vi "OME_coMD.vi"() -> ()   [LabVIEW 2012]
doc: "SciScan 1.2 160622"
uses:
  Macro Module/MacroGUI Module/Custom Controls and Typedefs/Cancel Settings.ctl
  Macro Module/MacroGUI Module/Custom Controls and Typedefs/Confirm Settings.ctl
  Custom Controls and Typedefs/Channel Parameters Cluster.ctl
  Custom Controls and Typedefs/Experiment and Experimenter.ctl
  Custom Controls and Typedefs/Objective Parameters Cluster.ctl
  Custom Controls and Typedefs/OME_MD_GUI control references.ctl
  CommonResource VIs/UI Control and Indicator properties_Commands.ctl
  SubVIs/FGV_ExclusionList_Manager_Commands.ctl
  CommonResource VIs/FormatTree&TableStyle_Commands.ctl
  GFG/GFGpathGet.vi
  <vilib>/xml/Close Reference(Node).vi
  <resource>/objmgr/DOMUserDefRef.rc
  <vilib>/xml/NI_XML.lvlib
  GFG/GFG library.lvlib
panel:
  in  "Objective Parameters":T1[](array[typedef])
  in  "Experiment Parameters":T2
  out "Parse Errors":string
  in  "Channel Parameters":T3[](array[typedef]) {"Excitation Wavelength" min=1e-07; "Emission Wavelength" min=1e-07}
  out "Selected Parameter Path":string caption="/OME/Experiment/ExperimenterRef/@ID"
  in  "Confirm":T4
  in  "Cancel":T5
  out "x-y":u32
  in  "Stop Button":bool
  in  "Refresh Button":bool
  in  "Param Value (Edit)":string caption="/OME/Experiment/ExperimenterRef/@ID"
  in  "XML 2D Array":string[][](array[string])
  in  "OME XML Parameters":string(tree)
  # "Experiment"
  # "Experimenter"
  # "Sample"
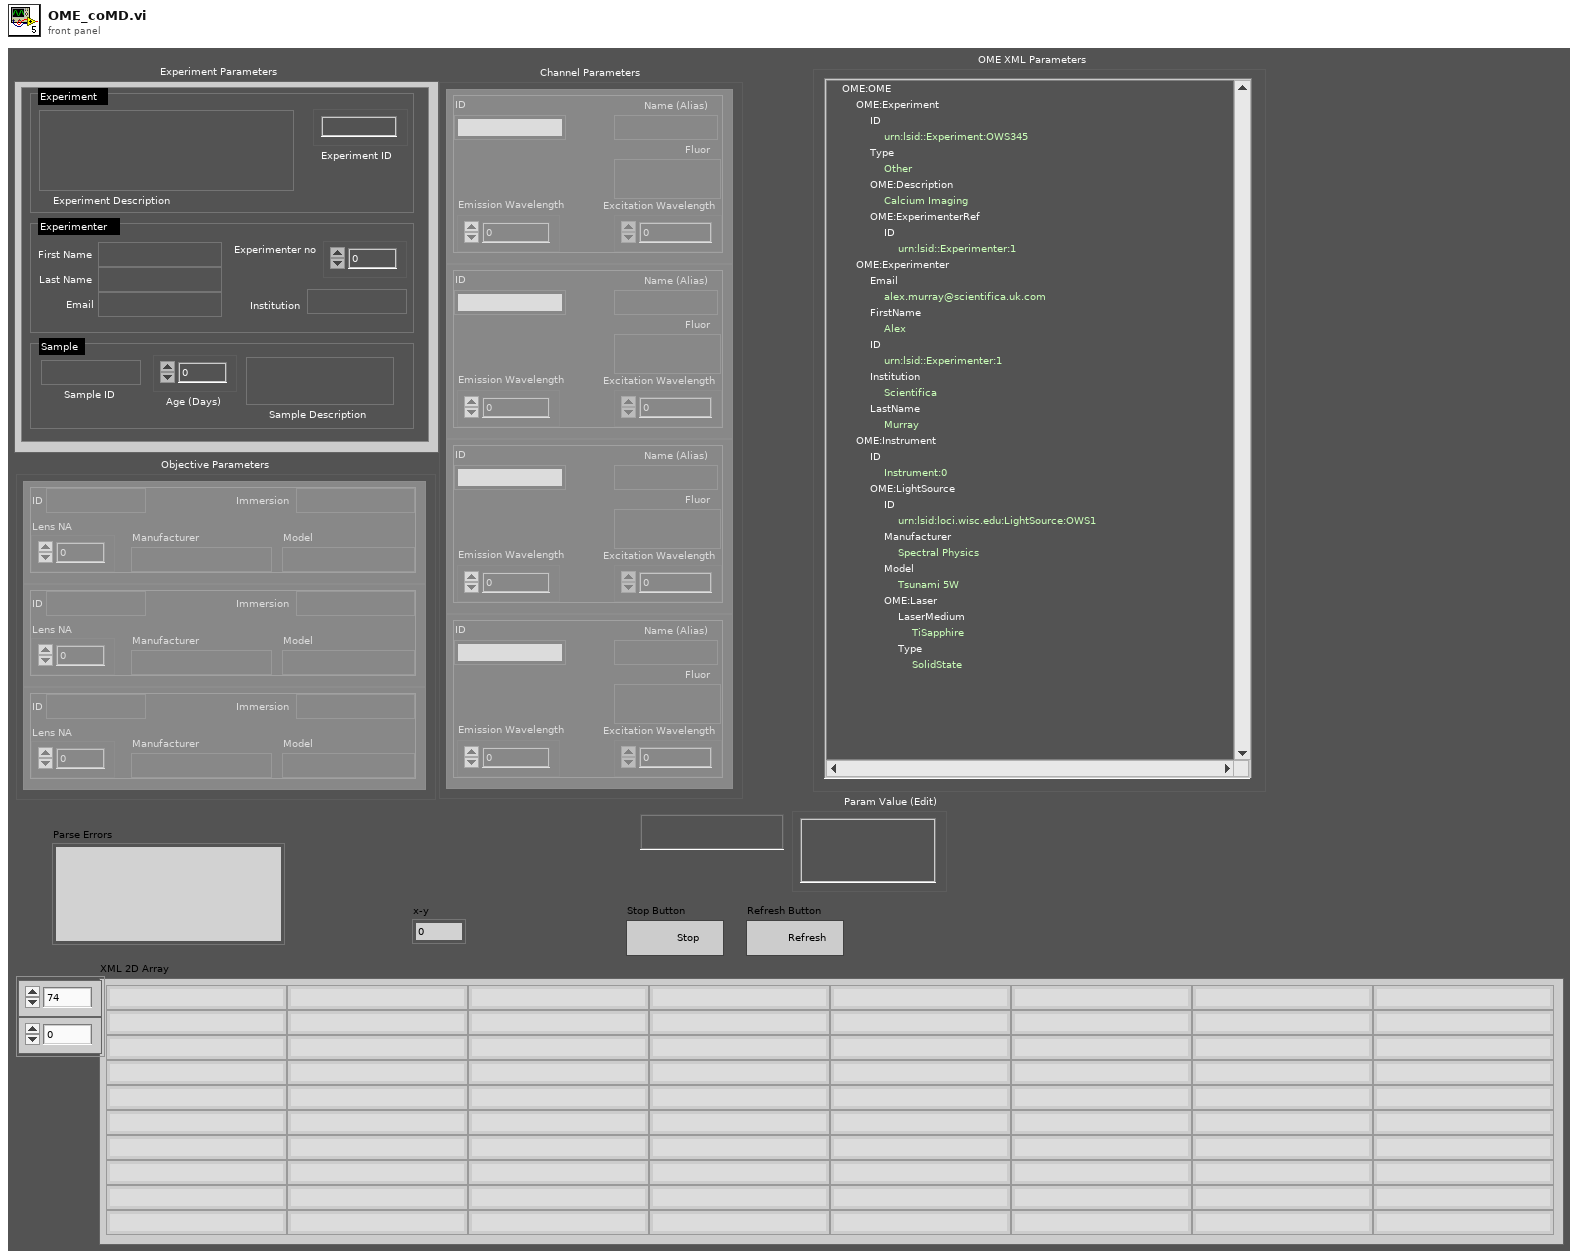
[diagram p1: front panel]
types:
  T1 = typedef "Objective Parameters Cluster.ctl" = cluster{"ID":string, "Immersion":string, "Lens NA":dbl, "Manufacturer":string, "Model":string}
  T2 = typedef "Experiment and Experimenter.ctl" = cluster{"Experimenter no":u32, "First Name":string, "Experiment ID":string, "urn:lsid: ":string, "Experiment Description":string, "Last Name":string, "Email":string, "Institution":string, "Sample ID":string, "Age (Days)":u32, "Sample Description":string}
  T3 = typedef "Channel Parameters Cluster.ctl" = cluster{"Name (Alias)":string, "ID":string, "Fluor":string, "Colour (RGBA encoded)":i32, "Emission Wavelength":dbl, "Excitation Wavelength":dbl}
  T4 = typedef "Confirm Settings.ctl" = bool
  T5 = typedef "Cancel Settings.ctl" = bool
  T6 = typedef "FGV_ExclusionList_Manager_Commands.ctl" = enum16{"Initialize(ReadCSV)", "Get", "CategorizePaths"}
  T7 = typedef "UI Control and Indicator properties_Commands.ctl" = enum16{"Enable", "Disable", "Disable and Grey", "Make Visible", "Make Invisible"}
  T8 = typedef "OME_MD_GUI control references.ctl" = cluster{"2D Array":refnum<vi>, "XML Tree":refnum<vi>, "Param Value":refnum<vi>, "Cancel":refnum<vi>, "Confirm":refnum<vi>, "Param Path":refnum<vi>, "Objective Parameters":refnum<vi>, "Experiment and Experimenter Details":refnum<vi>, "Channel Parameters":refnum<vi>}
  T9 = typedef "FormatTree&TableStyle_Commands.ctl" = enum16{"Colour Row", "Uncolour Row", "Bold Row", "Unbold Row", "Clear", "UpdateVisibleRows"}
  T10 = enum32{"Invalid", "Standard", "Closed", "Hidden", "Minimized", "Maximized"}
  T11 = typedef "eventvkey.ctl" = enum16{"ASCII", "Enter", "Return", "Shift", "Ctrl", "Alt", "Cmd", "Opt", "Caps", "NumLock", "Clear", "Break", "Up", "Down", "Left", "Right", "Insert", "Delete", "Home", "End", "PageUp", "PageDown", "Escape", "Help", "Pause", "ScrollLock", "F1", "F2", "F3", "F4", "F5", "F6", "F7", "F8", "F9", "F10", "F11", "F12", "F13", "F14", "F15", "F16", "F17", "F18", "F19", "F20", "F21", "F22", "F23", "F24", "Play", "VolumeUp", "VolumeDown", "Mute", "Two Byte Char"}
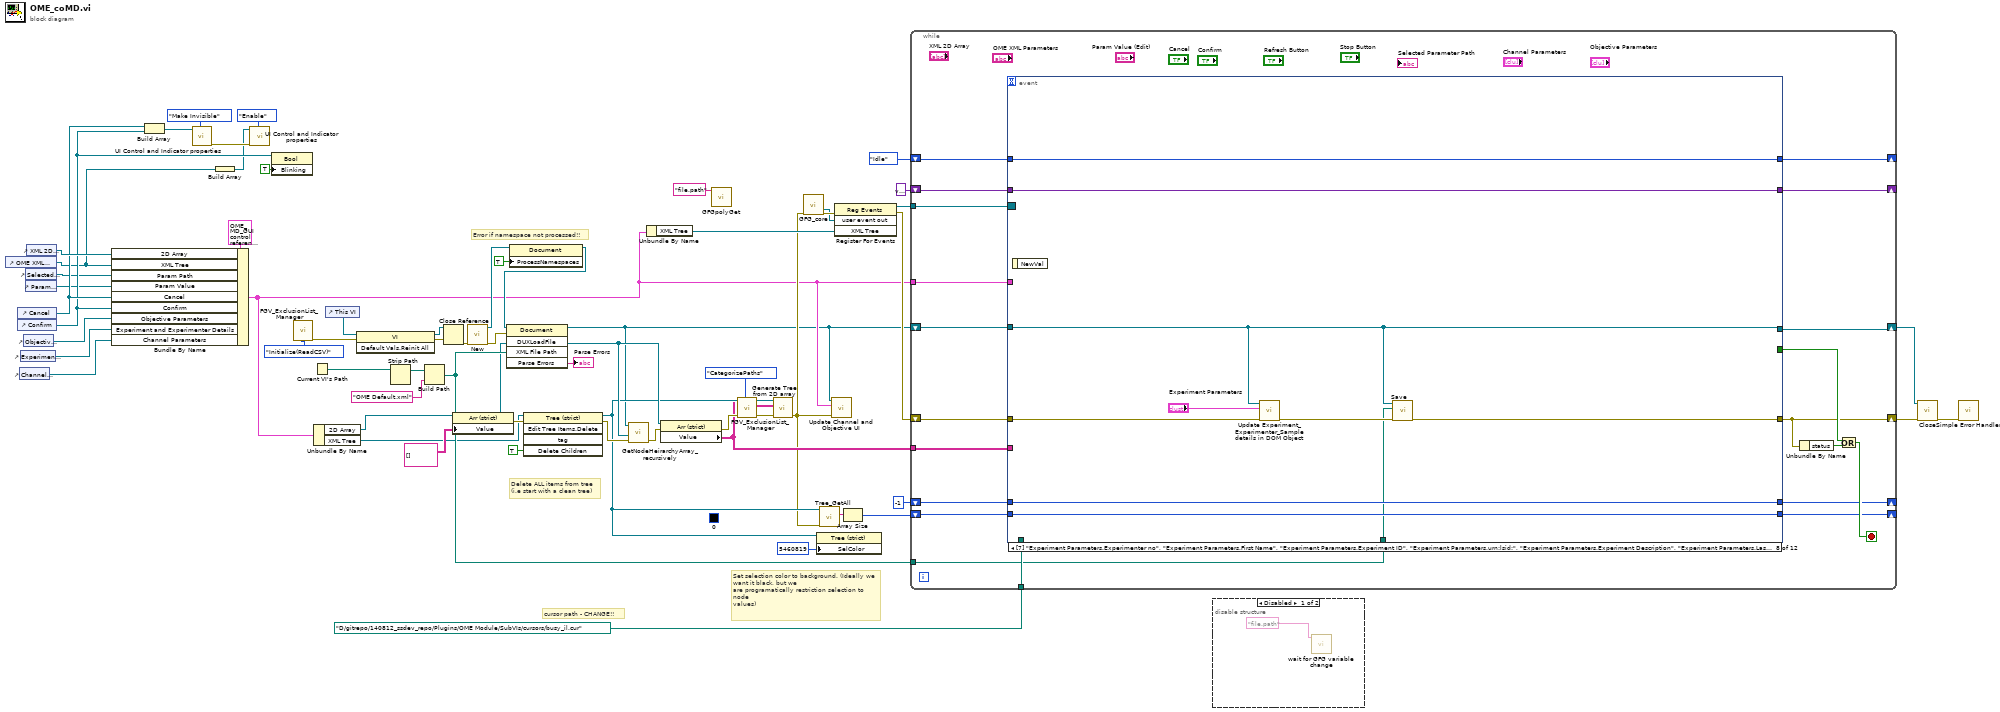
[diagram p0: block diagram]
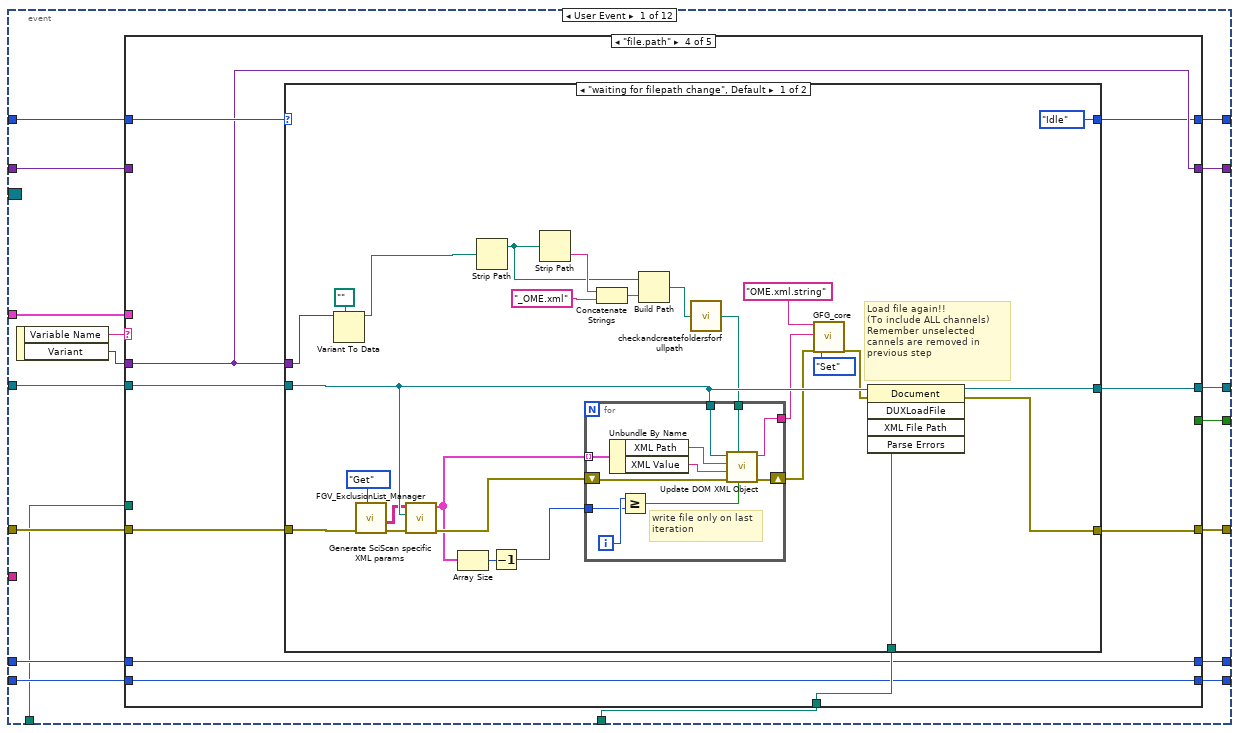
[diagram p3: hidden frame]
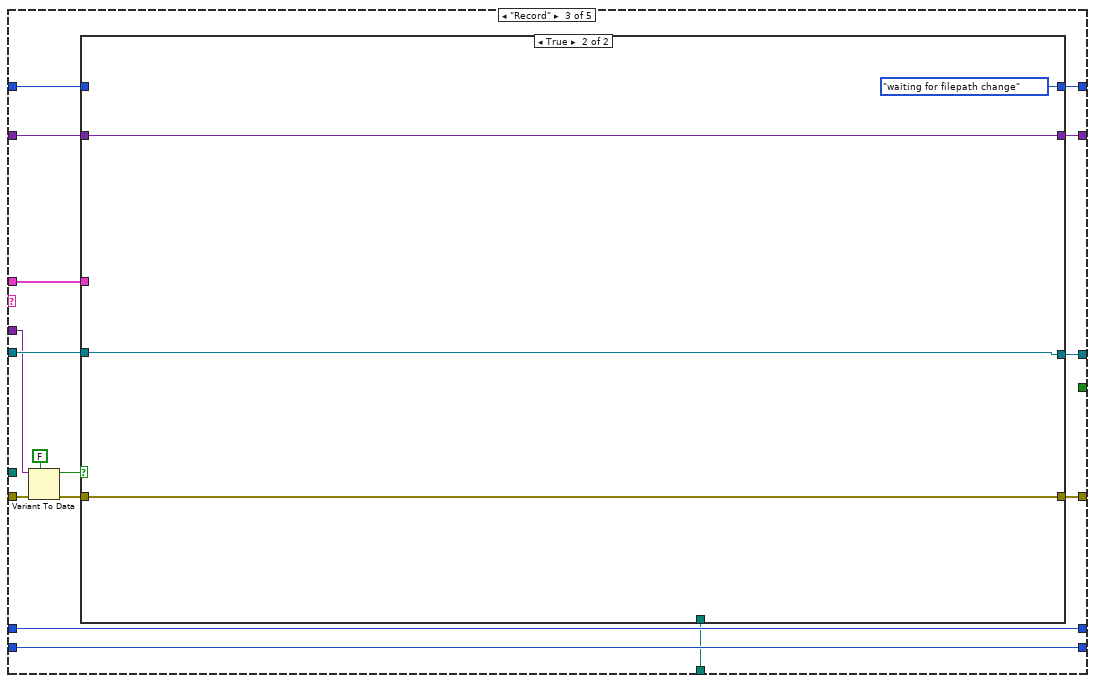
[diagram p6: hidden frame]
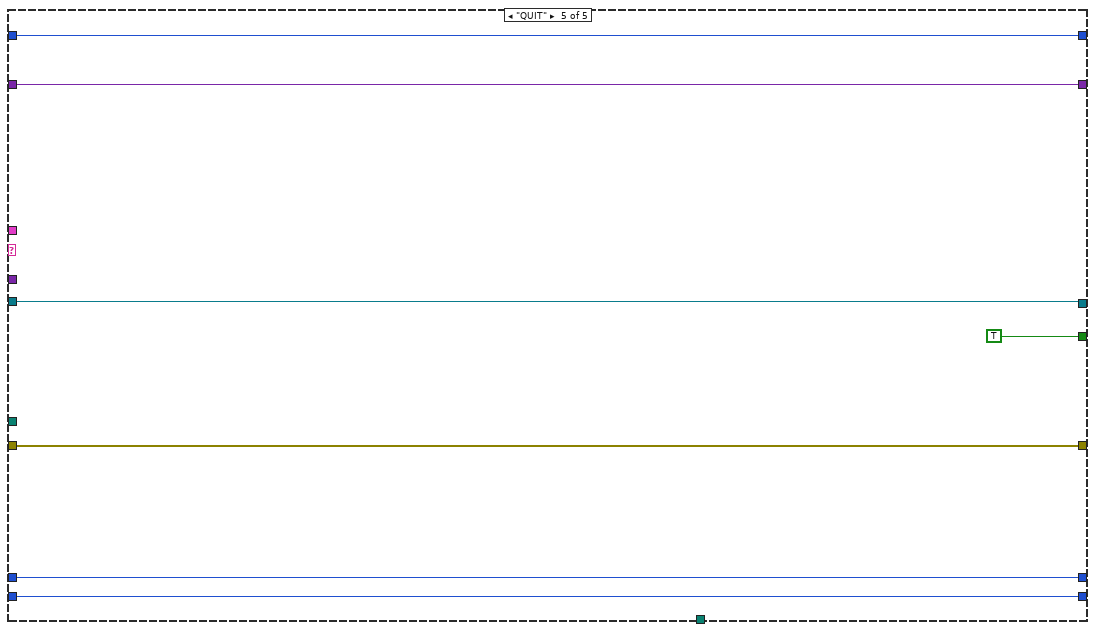
[diagram p9: hidden frame]
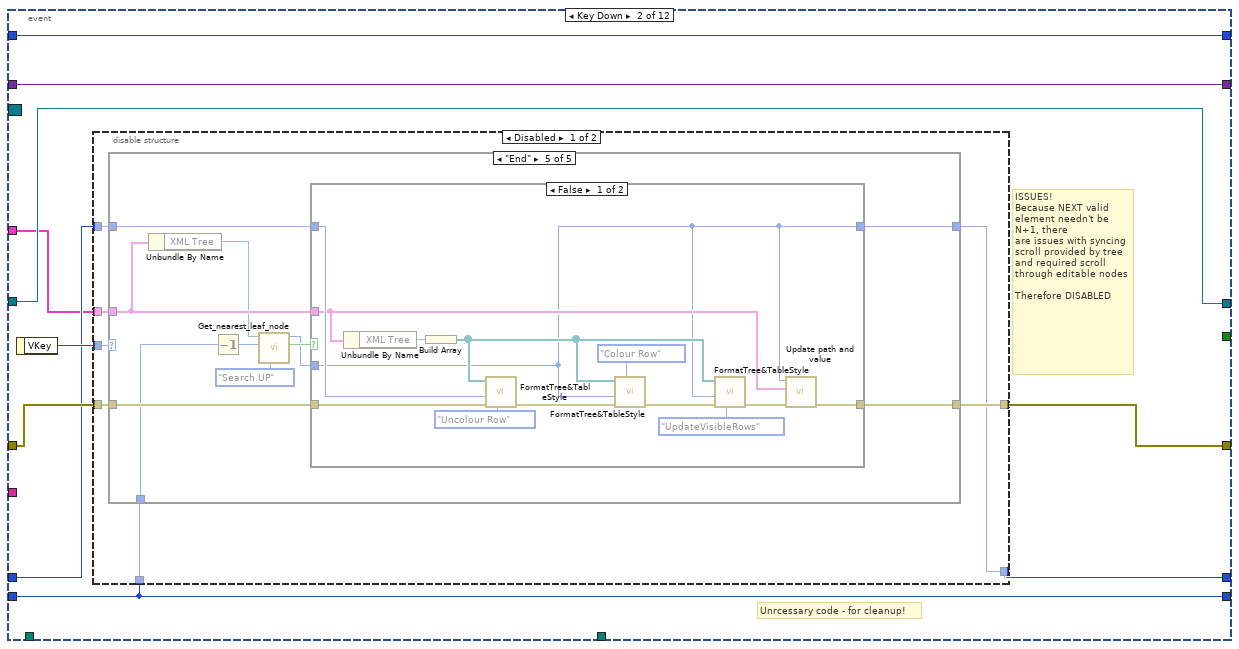
[diagram p10: hidden frame]
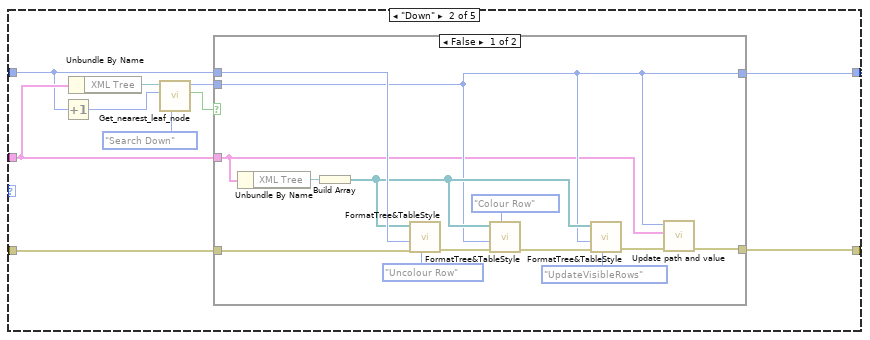
[diagram p12: hidden frame]
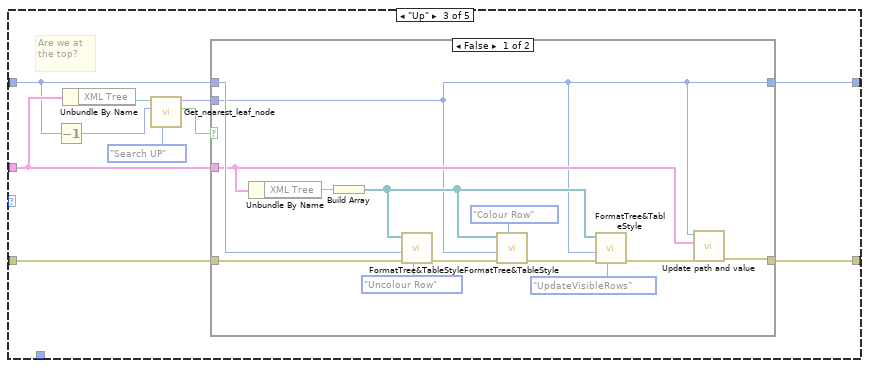
[diagram p14: hidden frame]
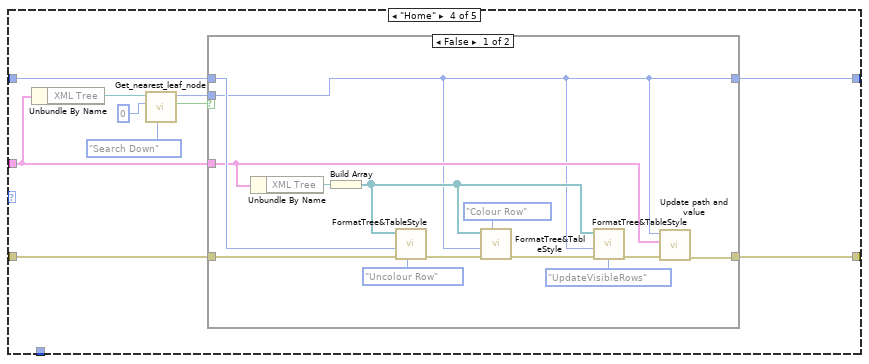
[diagram p16: hidden frame]
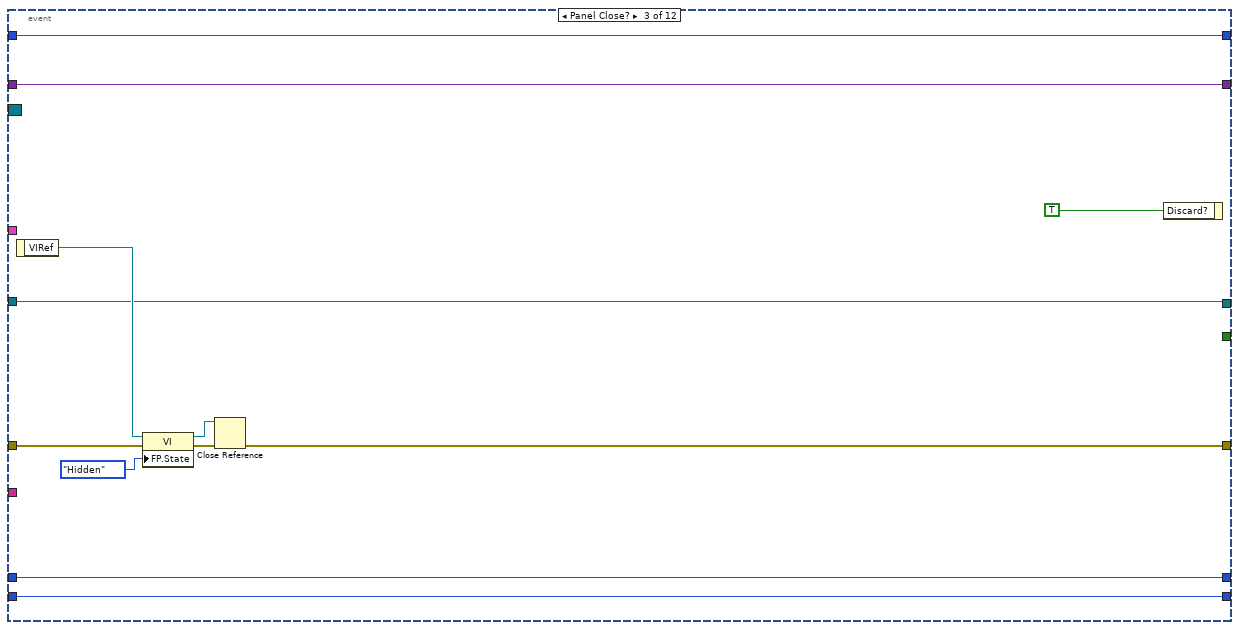
[diagram p20: hidden frame]
diagram:
  (unwired) u32 0
  # "Error if namespace not processed!!"
  # "cursor path - CHANGE!!"
  # "Set selection color to background. (Ideally we want it black, but we\nare programatically restriction selection to node\nvalues)"
  # "Delete ALL items from tree\n(i.e start with a clean tree)"
  n1 = control-ref of="OME XML Parameters"() -> (w33:refnum<vi>)
  n2 = control-ref of="Cancel"() -> (w38:refnum<vi>)
  n3 = control-ref of="Confirm"() -> (w37:refnum<vi>)
  n4 = control-ref of="Channel Parameters"() -> (w8:refnum<vi>)
  n5 = control-ref of="Experiment Parameters"() -> (w4:refnum<vi>)
  n6 = control-ref of="Objective Parameters"() -> (w9:refnum<vi>)
  n7 = control-ref of="Selected Parameter Path"() -> (w28:refnum<vi>)
  n8 = control-ref of="Param Value (Edit)"() -> (w27:refnum<vi>)
  n9 = control-ref of="XML 2D Array"() -> (w41:refnum<vi>)
  n10 = Bundle By Name(cluster=T8 {"2D Array"=refnum, "XML Tree"=refnum, "Param Value"=refnum, "Cancel"=refnum, "Confirm"=refnum, "Param Path"=refnum, "Objective Parameters"=refnum, "Experiment and Experimenter Details"=refnum, "Channel Parameters"=refnum} ("OME_MD_GUI control references"), "2D Array"=w41, "XML Tree"=w33, "Param Path"=w28, "Param Value"=w27, "Cancel"=w38, "Confirm"=w37, "Objective Parameters"=w9, "Experiment and Experimenter Details"=w4, "Channel Parameters"=w8) -> (w6:T8)
  n11 = Build Array(w38, w37) -> (w39:refnum<vi>[])
  n12 = call "UI Control and Indicator properties.vi"("Enable Command"=UI_Control_and_Indicator_properties_Commands."Make Invisible", "Control Refnums"=w39) -> ("Error Out"=w35:errorcluster)  [unwired: 9 in]
  n13 = Build Array(w33) -> (w32:refnum<vi>[])
  n14 = call "UI Control and Indicator properties.vi"("Enable Command"=UI_Control_and_Indicator_properties_Commands."Enable", "Error In"=w35, "Control Refnums"=w32) -> ()  [unwired: 8 in, 1 out]
  n15 = property class="Bool"(reference=w37, "Blinking"=TRUE) -> ()  [unwired: 1 in, 2 out]
  n16 = call "FGV_ExclusionList_Manager.vi"("Actions"=enum16{"Initialize(ReadCSV)", "Get"}."Initialize(ReadCSV)") -> ("error out"=w21:errorcluster)  [unwired: 5 in, 5 out]
  n17 = Current VI's Path() -> (path=w58:path)
  n18 = Unbundle By Name(w6) -> ("2D Array"=w30:refnum<vi>, "XML Tree"=w29:refnum<vi>)
  n19 = control-ref of="This VI"() -> (w50:refnum<vi>)
  n20 = invoke class="VI" method="Default Vals.Reinit All"(reference=w50, error in=w21) -> (reference out=w48:refnum<vi>, error out=w49:errorcluster)  [unwired: 1 in, 1 out]
  n21 = Strip Path(path=w58) -> (stripped path=w57:path)  [unwired: 1 out]
  n22 = Build Path(base path=w57, name or relative path="OME Default.xml") -> (appended path=w31:path)
  n23 = Close Reference(reference=w48, error in (no error)=w49) -> (error out=w47:errorcluster)
  n24 = property class="Arr (strict)"(reference=w30, "Value"=string[][] []) -> (error out=w46:errorcluster)  [unwired: 1 in, 1 out]
  n25 = call <vilib>:"New.vi"("error in (no error)"=w47) -> ("error out"=w59:errorcluster, "DOM document out"=w11:refnum<k20>)  [unwired: 7 in]
  n26 = property class="Document"(reference=w11, "ProcessNamespaces"=TRUE ("Process Namespaces")) -> (reference out=w10:refnum<k20>)  [unwired: 1 in, 1 out]
  n27 = invoke class="Document" method="DUXLoadFile"(reference=w10, error in=w59, "XML File Path"=w31) -> (reference out=w5:refnum<k20>, "Parse Errors"=→"Parse Errors":string)  [unwired: 2 in, 3 out]
  n28 = invoke class="Tree (strict)" method="Edit Tree Items.Delete"(reference=w29, error in=w46, "Delete Children"=TRUE ("Delete Children?")) -> (reference out=w26:refnum<vi>, error out=w44:errorcluster)  [unwired: 2 in, 3 out]
  n29 = call "GetNodeHeirarchyArray_recursively.vi"("error in (no error)"=w44, "2D Array_All Paths"=w30, "Node IN"=w5) -> ("error out"=w43:errorcluster)  [unwired: 8 in]
  n30 = Unbundle By Name(w6) -> ("XML Tree"=w23:refnum<vi>)
  n31 = property class="Arr (strict)"(reference=w30, error in=w43) -> (error out=w20:errorcluster, "Value"=w19:string[][])  [unwired: 1 out]
  n32 = call-poly "GFGpolyGet.vi"("Variable Name in"="file.path") -> ()  [unwired: 8 in, 3 out]
  n33 = call "FGV_ExclusionList_Manager.vi"("Actions"=FGV_ExclusionList_Manager_Commands."CategorizePaths", "error in (no error)"=w20, "XML 2D Array"=w19) -> ("error out"=w17:errorcluster, "To Include"=w16:string[][])  [unwired: 3 in, 4 out]
  n34 = call "Generate Tree from 2D array.vi"("error in (no error)"=w17, "XML 2D Array"=w16, "Tree Refnum"=w26) -> ("error out"=w7:errorcluster)  [unwired: 8 in]
  n35 = call "GFG_core.vi"("error in (no error)"=w7) -> ("user event out"=w62:refnum<user-event>, "error out"=w63:errorcluster)  [unwired: 12 in, 5 out]
  n36 = property class="Tree (strict)"(reference=w26, "SelColor"=u32 5460819 ("Active Cell:Cell Background Color")) -> ()  [unwired: 1 in, 2 out]
  n37 = call "Tree_GetAll.vi"("Error In"=w7, "Tree Refnum IN"=w26) -> ("Tags"=w25:string[])  [unwired: 6 in, 3 out]
  n38 = call "Update Channel and Objective UI .vi"("error in (no error)"=w7, "OME_MD_GUI control references"=w6, "DOM document IN"=w5) -> ()  [unwired: 7 in, 2 out]
  n39 = register-events(error in=w63, w62, w23) -> (reference out=w61:refnum<event-registration>, error out=w60:errorcluster)  [unwired: 1 in]
  n40 = Array Size(array=w25) -> (size(s)=w24:i32)
  n41 = while {
    tunnel: w61 -> [w83]
    shift-right: [w78] -> w52
    shift-left: w60 -> [w82]
    shift-right: [w75] -> _
    shift-left: w24 -> [w76]
    shift-right: [w73] -> _
    shift-left: -1 ("Number of Rows") -> [w74]
    tunnel: path "D:/gitrepo/140812_ssdev_repo/Plugins/OME Module/SubVIs/cursors/busy_il.cur" ("cursor file") -> [w72]
    tunnel: w6 -> [w70]
    tunnel: w19 -> [w69]
    tunnel: w31 -> [w68]
    shift-right: [w71] -> w15
    shift-left: w5 -> [w77]
    shift-right: [w65] -> _
    shift-left: variant ("Variant") -> [w67]
    shift-right: [w64] -> _
    shift-left: enum16{"waiting for filepath change", "Idle"}."Idle" -> [w66]
    stop <- w79 stop-if-true
    n42 = event shown="[7] \"Experiment Parameters.Experimenter no\", \"Experiment Parameters.First Name\", \"Experiment Parameters.Experiment ID\", \"Experiment Parameters.urn:lsid:\", \"Experiment Parameters.Experiment Description\", \"Experiment Parameters.Last Name\", \"Experiment Parameters.Email\", \"Experiment Parameters.Institution\", \"Experiment Parameters.Sample ID\", \"Experiment Parameters.Age (Days)\", \"Experiment Parameters.Sample Description\": Value Change" {
      selector: w83 -> [_ _ _ _ _ _ _ _ _ _ _ _]
      dyn-events: _ -> [_ _ _ _ _ _ _ _ _ _ _ _]
      timeout: _ -> [_ _ _ _ _ _ _ _ _ _ _ _]
      tunnel: [w100 _ _ TRUE _ _ _ _ _ _ _ _] -> w80
      tunnel: w82 -> [w99 w205 w325 w336 w354 w405 w416 w445 _ w495 w528 w563]
      tunnel: [w95 w202 w324 w336 w352 w396 w415 w449 w455 w493 w524 w559] -> w78
      tunnel: w77 -> [w96 w201 w320 w333 w344 w407 w418 w448 w457 w503 w507 w552]
      tunnel: w76 -> [w93 w200 w322 w335 w343 w409 w422 w451 w462 w504 w537 _]
      tunnel: [w98 w200 w322 w335 w343 w409 w422 w451 w462 w504 w537 w553] -> w75
      tunnel: w74 -> [w94 w203 w321 w334 w353 w408 w421 w450 w461 w487 w518 _]
      tunnel: [w97 w198 w321 w334 w351 w408 w421 w450 w461 w487 w518 w554] -> w73
      tunnel: w72 -> [w92 _ _ _ _ _ _ _ _ _ _ w558]
      tunnel: [w88 w201 w320 w333 w344 w407 w418 w448 w457 w503 w507 w552] -> w71
      tunnel: w70 -> [w90 w199 _ _ w342 w404 _ _ _ w494 w530 w542]
      tunnel: w69 -> [_ _ _ _ _ _ _ _ _ _ _ _]
      tunnel: w68 -> [w89 _ _ _ _ _ w417 w446 w458 _ w512 _]
      tunnel: w67 -> [w91 w196 w318 w330 w337 w394 w410 w443 w452 w485 w505 w538]
      tunnel: w66 -> [w86 w197 w319 w331 w338 w395 w411 w444 w453 w486 w506 w539]
      tunnel: [w85 w196 w318 w330 w337 w394 w410 w443 w452 w485 w505 w538] -> w65
      tunnel: [w84 w197 w319 w331 w338 w395 w411 w444 w453 w486 w506 w539] -> w64
      event User Event {
        n43 = event-data() -> ("Variable Name"=w101:string, "Variant"=w87:variant)  [unwired: 1 in]
        n44 = case shown="\"file.path\"" w101 {
          tunnel: [_ _ _ _ TRUE] -> w100
          tunnel: w99 -> [w105 w111 w121 w141 w192]
          tunnel: [w106 w112 w127 w138 w193] -> w98
          tunnel: [w107 w113 w128 w139 w194] -> w97
          tunnel: w96 -> [w104 w110 w129 w144 w191]
          tunnel: [w105 w111 w126 w142 w192] -> w95
          tunnel: w94 -> [w107 w113 w128 w139 w194]
          tunnel: w93 -> [w106 w112 w127 w138 w193]
          tunnel: w92 -> [_ _ _ _ _]
          tunnel: w91 -> [w103 w109 w125 _ w190]
          tunnel: w87 -> [_ _ w124 w146 _]
          tunnel: w90 -> [_ _ w119 _ _]
          tunnel: w89 -> [_ _ w118 w140 _]
          tunnel: [w104 w110 w117 w143 w191] -> w88
          tunnel: w86 -> [w102 w108 w116 w147 w189]
          tunnel: [w103 w109 w115 w146 w190] -> w85
          tunnel: [w102 w108 w114 w145 w189] -> w84
          frame Default {
          }
          frame "OME_MD_first_launch" {
          }
          frame "Record" {
            n45 = Variant To Data(error in=w121, type=FALSE, Variant=w124) -> (data=w122:bool, error out=w120:errorcluster)
            n46 = case shown="True" w122 {
              tunnel: w120 -> [w133 w136]
              tunnel: w129 -> [w132 w137]
              tunnel: [w133 w136] -> w126
              tunnel: w125 -> [w131 w135]
              tunnel: w119 -> [_ _]
              tunnel: w118 -> [_ _]
              tunnel: [w132 w137] -> w117
              tunnel: w116 -> [w130 _]
              tunnel: [w131 w135] -> w115
              tunnel: [w130 enum16{"waiting for filepath change", "Idle"}."waiting for filepath change"] -> w114
              frame False {
              }
              frame True {
              }
            }
          }
          frame "file.path" {
            n47 = case shown="\"waiting for filepath change\", Default" w147 {
              selector: w147 -> [_ w188]
              tunnel: w146 -> [w152 _]
              tunnel: [enum16{"waiting for filepath change", "Idle"}."Idle" w188] -> w145
              tunnel: w144 -> [w174 w187]
              tunnel: [w173 w187] -> w143
              tunnel: [w148 w186] -> w142
              tunnel: w141 -> [w172 w186]
              tunnel: w140 -> [w149 _]
              frame "waiting for filepath change", Default {
                # "Load file again!!\n(To include ALL channels)\nRemember unselected cannels are removed in previous step"
                n48 = Variant To Data(type=path "", Variant=w152) -> (data=w151:path)  [unwired: 1 in, 1 out]
                n49 = call "FGV_ExclusionList_Manager.vi"("Actions"=FGV_ExclusionList_Manager_Commands."Get", "error in (no error)"=w172) -> ("error out"=w160:errorcluster, "To Exclude"=w159:string[][])  [unwired: 4 in, 4 out]
                n50 = call "Generate SciScan specific XML params.vi"("error in (no error)"=w160, "DOM document IN"=w174, "Non-Tree elements 2D array IN"=w159) -> ("error out"=w162:errorcluster, "Path-Value pairs Array"=w161:cluster{"XML Path":string, "XML Value":string}[])  [unwired: 7 in]
                n51 = Array Size(array=w161) -> (size(s)=w169:i32)
                n52 = Strip Path(path=w151) -> (stripped path=w164:path)  [unwired: 1 out]
                n53 = Decrement(x=w169) -> (x-1=w168:i32)
                n54 = Strip Path(path=w164) -> (name=w165:string)  [unwired: 1 out]
                n55 = Concatenate Strings(w165, "_OME.xml" ("string")) -> (w166:string)
                n56 = Build Path(base path=w164, name or relative path=w166) -> (appended path=w158:path)
                n57 = call "checkandcreatefoldersforfullpath.vi"("Path IN"=w158) -> ("Path OUT"=w157:path)  [unwired: 4 in]
                n58 = for {
                  tunnel: w174 -> [w185]
                  tunnel: w157 -> [w184]
                  tunnel: w161 -> [w179] mode=indexing
                  tunnel: w168 -> [w182]
                  shift-right: [w176] -> w171
                  shift-left: w162 -> [w180]
                  tunnel: [w175] -> w163
                  i -> [w183]
                  # "write file only on last\niteration"
                  n59 = Unbundle By Name(w179) -> ("XML Path"=w178:string, "XML Value"=w177:string)
                  n60 = Greater Or Equal?(x=w183, y=w182) -> (x >= y?=w181:bool)
                  n61 = call "Update DOM XML Object.vi"("Write to File?"=w181, "XML File Path"=w184, "error in (no error)"=w180, "New Value (String)"=w177, "XPath expression to node"=w178, "DOM Refnum (XML Document)"=w185) -> ("error out"=w176:errorcluster, "XML string out"=w175:string)  [unwired: 4 in]
                }
                n62 = call "GFG_core.vi"("Variable Name in"="OME.xml.string", "Variant in"=w163, "error in (no error)"=w171, "Action"=enum16{"Init", "Set", "Get", "Clear"}."Set") -> ("error out"=w156:errorcluster)  [unwired: 9 in, 6 out]
                n63 = invoke class="Document" method="DUXLoadFile"(reference=w174, error in=w156, "XML File Path"=w149) -> (reference out=w173:refnum<k20>, error out=w148:errorcluster)  [unwired: 2 in, 3 out]
              }
              frame "Idle" {
              }
            }
          }
          frame "QUIT" {
          }
        }
      }
      event Key Down {
        # "Unrcessary code - for cleanup!"
        # "ISSUES!\nBecause NEXT valid element needn't be N+1, there\nare issues with syncing scroll provided by tree and required scroll through editable nodes\n\nTherefore DISABLED"
        n64 = event-data() -> ("VKey"=w204:T11)  [unwired: 1 in]
        n65 = disable-structure shown="Disabled" {
          disable-tunnel: w205 -> [w212 w316]
          disable-tunnel: w204 -> [w211 _]
          disable-tunnel: w203 -> [w210 w317]
          disable-tunnel: [w209 w316] -> w202
          disable-tunnel: w200 -> [w208 _]
          disable-tunnel: w199 -> [w207 _]
          disable-tunnel: [w206 w317] -> w198
          frame Disabled {
            n66 = case shown="\"End\"" w211 {
              tunnel: w212 -> [w214 w224 w249 w271 w297]
              tunnel: [w214 w222 w248 w272 w298] -> w209
              tunnel: w207 -> [_ w220 w246 w269 w293]
              tunnel: w210 -> [w213 w215 w243 w274 w300]
              tunnel: [w213 w223 w247 w273 w299] -> w206
              tunnel: w208 -> [_ _ _ _ w296]
              frame "ASCII", Default {
              }
              frame "Down" {
                n67 = Increment(x=w215) -> (x+1=w218:i32)
                n68 = Unbundle By Name(w220) -> ("XML Tree"=w219:refnum<vi>)
                n69 = call "Get_nearest_leaf_node.vi"("Enum"=enum16{"Search UP", "Search Down"}."Search Down", "Row Number"=w218, "Tree Refnum"=w219) -> ("NOT Found Error"=w217:bool, "Leaf Row Number OUT (Check if no error)"=w216:i32)  [unwired: 7 in]
                n70 = case shown="False" w217 {
                  tunnel: w220 -> [w225 _]
                  tunnel: w224 -> [w236 w238]
                  tunnel: w215 -> [w235 w239]
                  tunnel: [w226 w239] -> w223
                  tunnel: [w228 w238] -> w222
                  tunnel: w216 -> [w226 _]
                  frame False {
                    n71 = Unbundle By Name(w225) -> ("XML Tree"=w230:refnum<vi>)
                    n72 = Build Array(w230) -> (w229:refnum<vi>[])
                    n73 = call "FormatTree&TableStyle.vi"("Format Command"=FormatTree&TableStyle_Commands."Uncolour Row", "Error In"=w236, "Row Index"=w235, "Array of Tree references"=w229) -> ("Error Out"=w233:errorcluster)  [unwired: 7 in]
                    n74 = call "FormatTree&TableStyle.vi"("Format Command"=FormatTree&TableStyle_Commands."Colour Row", "Error In"=w233, "Row Index"=w226, "Array of Tree references"=w229) -> ("Error Out"=w231:errorcluster)  [unwired: 7 in]
                    n75 = call "FormatTree&TableStyle.vi"("Format Command"=FormatTree&TableStyle_Commands."UpdateVisibleRows", "Error In"=w231, "Row Index"=w226, "Array of Tree references"=w229) -> ("Error Out"=w227:errorcluster)  [unwired: 7 in]
                    n76 = call "Update path and value.vi"("error in (no error)"=w227, "OME_MD_GUI control references"=w225, "Row Index"=w226) -> ("error out"=w228:errorcluster)  [unwired: 8 in]
                  }
                  frame True {
                  }
                }
              }
              frame "Up" {
                # "Are we at the top?"
                n77 = Decrement(x=w243) -> (x-1=w242:i32)
                n78 = Unbundle By Name(w246) -> ("XML Tree"=w245:refnum<vi>)
                n79 = call "Get_nearest_leaf_node.vi"("Enum"=enum16{"Search UP", "Search Down"}."Search UP", "Row Number"=w242, "Tree Refnum"=w245) -> ("NOT Found Error"=w241:bool, "Leaf Row Number OUT (Check if no error)"=w240:i32)  [unwired: 7 in]
                n80 = case shown="False" w241 {
                  tunnel: w246 -> [w251 _]
                  tunnel: w249 -> [w261 w263]
                  tunnel: w243 -> [w260 w264]
                  tunnel: [w252 w263] -> w248
                  tunnel: [w250 w264] -> w247
                  tunnel: w240 -> [w250 _]
                  frame False {
                    n81 = Unbundle By Name(w251) -> ("XML Tree"=w257:refnum<vi>)
                    n82 = Build Array(w257) -> (w254:refnum<vi>[])
                    n83 = call "FormatTree&TableStyle.vi"("Format Command"=FormatTree&TableStyle_Commands."Uncolour Row", "Error In"=w261, "Row Index"=w260, "Array of Tree references"=w254) -> ("Error Out"=w258:errorcluster)  [unwired: 7 in]
                    n84 = call "FormatTree&TableStyle.vi"("Format Command"=FormatTree&TableStyle_Commands."Colour Row", "Error In"=w258, "Row Index"=w250, "Array of Tree references"=w254) -> ("Error Out"=w255:errorcluster)  [unwired: 7 in]
                    n85 = call "FormatTree&TableStyle.vi"("Format Command"=FormatTree&TableStyle_Commands."UpdateVisibleRows", "Error In"=w255, "Row Index"=w250, "Array of Tree references"=w254) -> ("Error Out"=w253:errorcluster)  [unwired: 7 in]
                    n86 = call "Update path and value.vi"("error in (no error)"=w253, "OME_MD_GUI control references"=w251, "Row Index"=w250) -> ("error out"=w252:errorcluster)  [unwired: 8 in]
                  }
                  frame True {
                  }
                }
              }
              frame "Home" {
                n87 = Unbundle By Name(w269) -> ("XML Tree"=w268:refnum<vi>)
                n88 = call "Get_nearest_leaf_node.vi"("Enum"=enum16{"Search UP", "Search Down"}."Search Down", "Row Number"=0 ("Index"), "Tree Refnum"=w268) -> ("NOT Found Error"=w266:bool, "Leaf Row Number OUT (Check if no error)"=w265:i32)  [unwired: 7 in]
                n89 = case shown="False" w266 {
                  tunnel: w269 -> [w276 _]
                  tunnel: w274 -> [w285 w289]
                  tunnel: w271 -> [w287 w288]
                  tunnel: [w275 w289] -> w273
                  tunnel: [w277 w288] -> w272
                  tunnel: w265 -> [w275 _]
                  frame False {
                    n90 = Unbundle By Name(w276) -> ("XML Tree"=w282:refnum<vi>)
                    n91 = Build Array(w282) -> (w279:refnum<vi>[])
                    n92 = call "FormatTree&TableStyle.vi"("Format Command"=FormatTree&TableStyle_Commands."Uncolour Row", "Error In"=w287, "Row Index"=w285, "Array of Tree references"=w279) -> ("Error Out"=w283:errorcluster)  [unwired: 7 in]
                    n93 = call "FormatTree&TableStyle.vi"("Format Command"=FormatTree&TableStyle_Commands."Colour Row", "Error In"=w283, "Row Index"=w275, "Array of Tree references"=w279) -> ("Error Out"=w280:errorcluster)  [unwired: 7 in]
                    n94 = call "FormatTree&TableStyle.vi"("Format Command"=FormatTree&TableStyle_Commands."UpdateVisibleRows", "Error In"=w280, "Row Index"=w275, "Array of Tree references"=w279) -> ("Error Out"=w278:errorcluster)  [unwired: 7 in]
                    n95 = call "Update path and value.vi"("error in (no error)"=w278, "OME_MD_GUI control references"=w276, "Row Index"=w275) -> ("error out"=w277:errorcluster)  [unwired: 8 in]
                  }
                  frame True {
                  }
                }
              }
              frame "End" {
                n96 = Unbundle By Name(w293) -> ("XML Tree"=w292:refnum<vi>)
                n97 = Decrement(x=w296) -> (x-1=w294:u32)
                n98 = call "Get_nearest_leaf_node.vi"("Enum"=enum16{"Search UP", "Search Down"}."Search UP", "Row Number"=w294, "Tree Refnum"=w292) -> ("NOT Found Error"=w291:bool, "Leaf Row Number OUT (Check if no error)"=w290:i32)  [unwired: 7 in]
                n99 = case shown="False" w291 {
                  tunnel: w293 -> [w302 _]
                  tunnel: w300 -> [w311 w315]
                  tunnel: w297 -> [w313 w314]
                  tunnel: [w301 w315] -> w299
                  tunnel: [w303 w314] -> w298
                  tunnel: w290 -> [w301 _]
                  frame False {
                    n100 = Unbundle By Name(w302) -> ("XML Tree"=w308:refnum<vi>)
                    n101 = Build Array(w308) -> (w305:refnum<vi>[])
                    n102 = call "FormatTree&TableStyle.vi"("Format Command"=FormatTree&TableStyle_Commands."Uncolour Row", "Error In"=w313, "Row Index"=w311, "Array of Tree references"=w305) -> ("Error Out"=w309:errorcluster)  [unwired: 7 in]
                    n103 = call "FormatTree&TableStyle.vi"("Format Command"=FormatTree&TableStyle_Commands."Colour Row", "Error In"=w309, "Row Index"=w301, "Array of Tree references"=w305) -> ("Error Out"=w306:errorcluster)  [unwired: 7 in]
                    n104 = call "FormatTree&TableStyle.vi"("Format Command"=FormatTree&TableStyle_Commands."UpdateVisibleRows", "Error In"=w306, "Row Index"=w301, "Array of Tree references"=w305) -> ("Error Out"=w304:errorcluster)  [unwired: 7 in]
                    n105 = call "Update path and value.vi"("error in (no error)"=w304, "OME_MD_GUI control references"=w302, "Row Index"=w301) -> ("error out"=w303:errorcluster)  [unwired: 8 in]
                  }
                  frame True {
                  }
                }
              }
            }
          }
          frame Enabled {
          }
        }
      }
      event Panel Close? {
        n106 = event-data() -> ("VIRef"=w327:refnum<vi>)  [unwired: 1 in]
        n107 = property class="VI"(reference=w327, error in=w325, "FP.State"=T10."Hidden" ("Front Panel Window:State")) -> (reference out=w323:refnum<vi>, error out=w328:errorcluster)
        n108 = Close Reference(reference=w323, error in (no error)=w328) -> (error out=w324:errorcluster)
        n109 = event-data("Discard?"=TRUE) -> ()  [unwired: 1 in, 1 out]
      }
      event "Stop Button": Value Change {
        n110 = event-data() -> ()  [unwired: 1 in, 1 out]
      }
      event "OME XML Parameters": Mouse Down {
        # "Unrcessary code - for cleanup!"
        # "no children?"
        # "are there any elements?"
        # "Valid selection?"
        n111 = event-data() -> ()  [unwired: 1 in, 1 out]
        n112 = Unbundle By Name(w342) -> ("Param Path"=w339:refnum<vi>, "Param Value"=w341:refnum<vi>, "XML Tree"=w340:refnum<vi>)
        n113 = property class="Tree (strict)"(reference=w340, error in=w354) -> (error out=w350:errorcluster, "Value"=w345:string, "All Tags"=w357:string[])  [unwired: 1 out]
        n114 = Greater Or Equal To 0?(x=w343) -> (x >= 0?=w359:bool)
        n115 = Search 1D Array(1D array=w357, element=w345) -> (index of element=w356:i32)  [unwired: 1 in]
        n116 = Greater Or Equal To 0?(x=w356) -> (x >= 0?=w355:bool)
        n117 = invoke class="Tree (strict)" method="Navigate Tree.Get Child"(reference=w340, error in=w350, "Tag"=w345) -> (reference out=w348:refnum<vi>, error out=w346:errorcluster, "Navigate Tree:Get Child"=w349:string)  [unwired: 1 in, 1 out]
        n118 = Empty String/Path?(string/path=w349) -> (empty?=w347:bool)
        n119 = Compound Arithmetic op=AND(w359, w355, w347) -> (w358:bool)
        n120 = case shown="True" w358 {
          tunnel: w353 -> [w360 w384]
          tunnel: [w361 w365] -> w352
          tunnel: w346 -> [w361 w373]
          tunnel: w348 -> [_ w378]
          tunnel: w345 -> [_ w387]
          tunnel: [w360 w380] -> w351
          tunnel: w341 -> [_ w363]
          tunnel: w345 -> [_ w377]
          tunnel: w339 -> [_ w364]
          frame False {
          }
          frame True {
            # "Update the parameter path and value\nvalue"
            n121 = First Call?() -> (First Call?: T/F=w362:bool)
            n122 = case shown="True" w362 {
              tunnel: w364 -> [_ w393]
              tunnel: w363 -> [_ w392]
              frame False {
              }
              frame True {
                n123 = Build Array(w393, w392) -> (w390:refnum<vi>[])
                n124 = call "UI Control and Indicator properties.vi"("Enable Command"=UI_Control_and_Indicator_properties_Commands."Make Visible", "Control Refnums"=w390) -> ()  [unwired: 9 in, 1 out]
              }
            }
            n125 = invoke class="Tree (strict)" method="Navigate Tree.Get Path"(reference=w378, error in=w373, "tag"=w377) -> (reference out=w375:refnum<vi>, error out=w372:errorcluster, "Navigate Tree:Get Path"=w376:string[])  [unwired: 1 in, 1 out]
            n126 = Build Array(w378) -> (w381:refnum<vi>[])
            n127 = call "FormatTree&TableStyle.vi"("Format Command"=FormatTree&TableStyle_Commands."Uncolour Row", "Error In"=w373, "Row Index"=w384, "Array of Tree references"=w381) -> ("Error Out"=w386:errorcluster)  [unwired: 7 in]
            n128 = call "Tree_GetIndexFromTag.vi"("Error In"=w386, "Tag IN"=w387, "Tree Refnum IN"=w378) -> ("Error Out"=w389:errorcluster, "Index OUT"=w380:i32, "Tree Refnum OUT"=w388:refnum<vi>)  [unwired: 6 in]
            n129 = call "Tree_GetTextFromTag.vi"("Error In"=w372, "Tag IN"=w377, "Tree Refnum IN"=w375) -> ("Error Out"=w370:errorcluster, "String OUT"=w379:string)  [unwired: 6 in, 1 out]
            n130 = call "TreePath_to_XMLAttributePath.vi"("error in (no error)"=w372, "Tree Refnum"=w375, "Tree Path (Array)"=w376) -> ("error out"=w371:errorcluster, "XML Attribute path (String)"=w374:string)  [unwired: 6 in, 1 out]
            n131 = Close Reference(reference=w388, error in (no error)=w389) -> (error out=w382:errorcluster)
            n132 = property class="Str"(reference=w363, error in=w370, "Value"=w379) -> (error out=w369:errorcluster)  [unwired: 1 out]
            n133 = property class="Str"(reference=w364, error in=w371, "Value"=w374) -> (error out=w368:errorcluster)  [unwired: 1 out]
            n134 = call "FormatTree&TableStyle.vi"("Format Command"=FormatTree&TableStyle_Commands."Colour Row", "Error In"=w382, "Row Index"=w380, "Array of Tree references"=w381) -> ("Error Out"=w367:errorcluster)  [unwired: 7 in]
            n135 = Merge Errors(w369, w368) -> (w366:errorcluster)
            n136 = Merge Errors(w366, w367) -> (w365:errorcluster)
          }
        }
      }
      event "Param Value (Edit)": Value Change {
        n137 = event-data() -> ()  [unwired: 1 in, 1 out]
        n138 = Unbundle By Name(w404) -> ("XML Tree"=w399:refnum<vi>, "Cancel"=w403:refnum<vi>, "Confirm"=w402:refnum<vi>)
        n139 = Build Array(w403, w402) -> (w401:refnum<vi>[])
        n140 = Build Array(w399) -> (w398:refnum<vi>[])
        n141 = call "UI Control and Indicator properties.vi"("Enable Command"=UI_Control_and_Indicator_properties_Commands."Make Visible", "Error In"=w405, "Control Refnums"=w401) -> ("Error Out"=w397:errorcluster)  [unwired: 8 in]
        n142 = call "UI Control and Indicator properties.vi"("Enable Command"=UI_Control_and_Indicator_properties_Commands."Disable and Grey", "Error In"=w397, "Control Refnums"=w398) -> ("Error Out"=w396:errorcluster)  [unwired: 8 in]
      }
      event "Objective Parameters": Value Change {
        n143 = event-data() -> ("NewVal"=w414:T1[])  [unwired: 1 in]
        n144 = call "Update SciScan Objective Info with OME data.vi"("error in (no error)"=w416, "Objective Parameters"=w414) -> ("error out"=w413:errorcluster)  [unwired: 9 in]
        n145 = call <vilib>:"Get All Matched Nodes.vi"("XPath expression"="/OME:OME/OME:Instrument/OME:Objective", "node in"=w418) -> ("node result array"=w419:refnum<k20>[])  [unwired: 7 in, 2 out]
        n146 = for {
          tunnel: w414 -> [w437] mode=indexing
          tunnel: w419 -> [w424] mode=indexing
          shift-right: [w423] -> w412
          shift-left: w413 -> [w423]
          n147 = Unbundle By Name(w437) -> ("Immersion"=w434:string, "Lens NA"=w435:dbl, "Manufacturer"=w432:string, "Model"=w431:string)
          n148 = Number To Fractional String(number=w435, precision (6)=i16 2) -> (F-format string=w433:string)  [unwired: 2 in]
          n149 = Build Array("@Immersion" ("XPath expression"), "@LensNA" ("XPath expression"), "@Manufacturer" ("XPath expression"), "@Model" ("XPath expression")) -> (w425:string[])
          n150 = Build Array(w434, w433, w432, w431) -> (w426:string[])
          n151 = for {
            tunnel: w426 -> [w438] mode=indexing
            tunnel: w425 -> [w440] mode=indexing
            tunnel: w424 -> [w441]
            n152 = call <vilib>:"Get First Matched Node.vi"("XPath expression"=w440, "node in"=w441) -> ("node result"=w439:refnum<k20>)  [unwired: 7 in, 2 out]
            n153 = property class="Node"(reference=w439, "Value"=w438) -> ()  [unwired: 1 in, 2 out]
          }
        }
        n154 = call <vilib>:"Save.vi"("error in (no error)"=w412, "XML file path"=w417, "DOM document in"=w418) -> ("error out"=w415:errorcluster)  [unwired: 6 in, 2 out]
      }
      event Value Change {
        n155 = event-data() -> ()  [unwired: 1 in, 1 out]
        n156 = call "Update Experiment_Experimenter_Sample details in DOM Object.vi"("error in (no error)"=w445, "Experiment|_Experimenter_Sample_Cluster IN"="Experiment Parameters", "Refnum in"=w448) -> ("error out"=w447:errorcluster)  [unwired: 8 in]
        n157 = call <vilib>:"Save.vi"("error in (no error)"=w447, "XML file path"=w446, "DOM document in"=w448) -> ("error out"=w449:errorcluster)  [unwired: 6 in, 2 out]
      }
      event "Channel Parameters": Value Change {
        n158 = event-data() -> ("NewVal"=w460:T3[])  [unwired: 1 in]
        n159 = call <vilib>:"Get All Matched Nodes.vi"("XPath expression"="/OME:OME/OME:Image/OME:Pixels/OME:Channel", "node in"=w457) -> ("node result array"=w459:refnum<k20>[])  [unwired: 7 in, 2 out]
        n160 = for {
          tunnel: w460 -> [w478] mode=indexing
          tunnel: w459 -> [w479] mode=indexing
          tunnel: [w474] -> w456
          w473 = i16 12 ("precision (6)")
          (unwired) i16 2 ("precision (6)")
          n161 = Unbundle By Name(w478) -> ("Name (Alias)"=w469:string, "Fluor"=w468:string, "Colour (RGBA encoded)"=w476:i32, "Emission Wavelength"=w477:dbl, "Excitation Wavelength"=w475:dbl)
          n162 = Build Array("@Name" ("XPath expression"), "@Fluor" ("XPath expression"), "@EmissionWavelength" ("XPath expression"), "@ExcitationWavelength" ("XPath expression")) -> (w467:string[])
          n163 = Number To Fractional String(number=w477, precision (6)=w473) -> (F-format string=w470:string)  [unwired: 2 in]
          n164 = Number To Decimal String(number=w476) -> ()  [unwired: 1 in, 1 out]
          n165 = Number To Fractional String(number=w475, precision (6)=w473) -> (F-format string=w471:string)  [unwired: 2 in]
          n166 = Build Array(w469, w468, w470, w471) -> (w472:string[])
          n167 = for {
            tunnel: w472 -> [w481] mode=indexing
            tunnel: w467 -> [w483] mode=indexing
            tunnel: w479 -> [w484]
            tunnel: [w480] -> w474
            n168 = call <vilib>:"Get First Matched Node.vi"("XPath expression"=w483, "node in"=w484) -> ("node result"=w482:refnum<k20>)  [unwired: 7 in, 2 out]
            n169 = property class="Node"(reference=w482, "Value"=w481) -> (error out=w480:errorcluster)  [unwired: 1 in, 1 out]
          }
        }
        n170 = call <vilib>:"Save.vi"("error in (no error)"=w456, "XML file path"=w458, "DOM document in"=w457) -> ("error out"=w455:errorcluster)  [unwired: 6 in, 2 out]
      }
      event "Cancel": Value Change {
        # "Unrcessary code - for cleanup!"
        n171 = event-data() -> ()  [unwired: 1 in, 1 out]
        n172 = Unbundle By Name(w494) -> ("XML Tree"=w491:refnum<vi>, "Cancel"=w501:refnum<vi>, "Confirm"=w500:refnum<vi>, "Param Value"=w492:refnum<vi>)
        n173 = Build Array(w501, w500) -> (w499:refnum<vi>[])
        n174 = Build Array(w491) -> (w497:refnum<vi>[])
        n175 = call "UI Control and Indicator properties.vi"("Enable Command"=UI_Control_and_Indicator_properties_Commands."Make Invisible", "Error In"=w495, "Control Refnums"=w499) -> ("Error Out"=w496:errorcluster)  [unwired: 8 in]
        n176 = call "UI Control and Indicator properties.vi"("Enable Command"=UI_Control_and_Indicator_properties_Commands."Enable", "Error In"=w496, "Control Refnums"=w497) -> ("Error Out"=w490:errorcluster)  [unwired: 8 in]
        n177 = call "Tree_GetTag FromIndex.vi"("Error In"=w490, "Index IN"=w487, "Tree Refnum IN"=w491) -> ("Error Out"=w489:errorcluster, "Tag OUT"=w488:string)  [unwired: 6 in, 1 out]
        n178 = property class="Str"(reference=w492, error in=w489, "Value"=w488) -> (error out=w493:errorcluster)  [unwired: 1 out]
      }
      event "Confirm": Value Change {
        # "Unrcessary code - for cleanup!"
        # "If empty string,\nadd a '*'"
        # "Update the relevant parameter value in the DOM object; and \nthen write to XML file"
        # "Update Tree String"
        n179 = event-data() -> ()  [unwired: 1 in, 1 out]
        n180 = Unbundle By Name(w530) -> ("XML Tree"=w519:refnum<vi>, "Cancel"=w535:refnum<vi>, "Confirm"=w534:refnum<vi>, "Param Value"=w520:refnum<vi>)
        n181 = property class="Str"(reference=w520, error in=w528) -> (error out=w527:errorcluster, "Value"=w510:string)  [unwired: 1 out]
        n182 = Build Array(w535, w534) -> (w533:refnum<vi>[])
        n183 = call "UI Control and Indicator properties.vi"("Enable Command"=UI_Control_and_Indicator_properties_Commands."Make Invisible", "Error In"=w527, "Control Refnums"=w533) -> ("Error Out"=w514:errorcluster)  [unwired: 8 in]
        n184 = Build Array(w519) -> (w531:refnum<vi>[])
        n185 = call "Tree_GetTag FromIndex.vi"("Error In"=w514, "Index IN"=w518, "Tree Refnum IN"=w519) -> ("Error Out"=w515:errorcluster, "Tag OUT"=w517:string, "Tree Refnum OUT"=w516:refnum<vi>)  [unwired: 6 in]
        n186 = invoke class="Tree" method="Navigate Tree.Get Path"(reference=w516, error in=w515, "tag"=w517) -> (reference out=w526:refnum<vi>, error out=w513:errorcluster, "Navigate Tree:Get Path"=w529:string[])  [unwired: 1 in, 1 out]
        n187 = call "TreePath_to_XMLAttributePath.vi"("Tree Refnum"=w526, "Tree Path (Array)"=w529) -> ("XML Attribute path (String)"=w511:string)  [unwired: 7 in, 2 out]
        n188 = call "Update DOM XML Object.vi"("Write to File?"=TRUE, "XML File Path"=w512, "error in (no error)"=w513, "New Value (String)"=w510, "XPath expression to node"=w511, "DOM Refnum (XML Document)"=w507) -> ("error out"=w508:errorcluster)  [unwired: 4 in, 1 out]
        n189 = Empty String/Path?(string/path=w510) -> (empty?=w523:bool)
        n190 = call "UI Control and Indicator properties.vi"("Enable Command"=UI_Control_and_Indicator_properties_Commands."Enable", "Error In"=w508, "Control Refnums"=w531) -> ("Error Out"=w525:errorcluster)  [unwired: 8 in]
        n191 = Select(t="*", s=w523, f=w510) -> (s? t:f=w521:string)
        n192 = property class="Tree (strict)"(reference=w519, error in=w525, "Active Item Tag"=w517, "Cell String"=w521) -> (error out=w524:errorcluster)  [unwired: 1 out]
      }
      event "Refresh Button": Value Change {
        # "Unrcessary code - for cleanup!"
        n193 = event-data() -> ()  [unwired: 1 in, 1 out]
        n194 = Unbundle By Name(w542) -> ("2D Array"=w540:refnum<vi>, "XML Tree"=w541:refnum<vi>)
        n195 = call <vilib>:"Create Cursor From File.vi"("error in (no error)"=w563, "cursor file"=w558) -> ("error out"=w562:errorcluster, "cursor ID"=w561:refnum<k1>)  [unwired: 8 in]
        n196 = call <vilib>:"Set Busy.vi"("error in (no error)"=w562, "cursor ID"=w561) -> ("error out"=w551:errorcluster)  [unwired: 8 in, 1 out]
        n197 = invoke class="Tree (strict)" method="Edit Tree Items.Delete"(reference=w541, error in=w551) -> (error out=w550:errorcluster)  [unwired: 3 in, 4 out]
        n198 = call "GetNodeHeirarchyArray_recursively.vi"("error in (no error)"=w550, "2D Array_All Paths"=w540, "Node IN"=w552) -> ("error out"=w546:errorcluster)  [unwired: 8 in]
        n199 = flat-sequence {
          tunnel: w546 -> [_]
          tunnel: [w565] -> w549
          frame #0 {
            n200 = Tick Count (ms)() -> (millisecond timer value=w565:u32)
          }
        }
        n201 = property class="Arr (strict)"(reference=w540, error in=w546) -> (error out=w545:errorcluster, "Value"=w543:string[][])  [unwired: 1 out]
        n202 = call "Generate Tree from 2D array.vi"("error in (no error)"=w545, "XML 2D Array"=w543, "Tree Refnum"=w541) -> ("error out"=w544:errorcluster)  [unwired: 8 in]
        n203 = property class="Tree (strict)"(reference=w541, error in=w544) -> (error out=w560:errorcluster, "NumRows"=w553:u32)  [unwired: 1 out]
        n204 = flat-sequence {
          tunnel: w544 -> [_]
          tunnel: [w564] -> w548
          frame #0 {
            n205 = Tick Count (ms)() -> (millisecond timer value=w564:u32)
          }
        }
        n206 = call <vilib>:"Unset Busy.vi"("error in (no error)"=w560) -> ("error out"=w559:errorcluster)  [unwired: 10 in]
        n207 = Greater Or Equal To 0?(x=w553) -> (x >= 0?=w557:bool)
        n208 = Subtract(x=w548, y=w549) -> (x-y=→"x-y":u32)
        n209 = Select(t=0 ("Number of Rows"), s=w557, f=-1 ("Number of Rows")) -> (s? t:f=w554:i32)
      }
    }
    n210 = Unbundle By Name(w78) -> ("status"=w81:bool)
    n211 = Or(x=w80, y=w81) -> (x .or. y?=w79:bool)
  }
  n212 = disable-structure shown="Disabled" {
    frame Disabled {
      n213 = call "wait for GFG variable change.vi"("Variable Name in"="file.path") -> ("error in"=w567:errorcluster, "Initialization Value"=w568:variant)  [unwired: 8 in, 1 out]
    }
    frame Enabled {
    }
  }
  n214 = call-poly <vilib>:"Close.vi"("error in (no error)"=w52, "node"=w15) -> ("error out"=w51:errorcluster)  [unwired: 7 in]
  n215 = call <vilib>:"Simple Error Handler.vi"("error in (no error)"=w51) -> ()  [unwired: 4 in, 5 out]
